vi "writeU32FIFO.vi"(8 "error in (no error)":errorcluster, 9 "Timeout":i32, 10 "Data":u32[](array[numeric]), 11 "IWriteU32FIFO in":refnum<class "IWriteU32FIFO.lvclass">) -> (0 "error out":errorcluster, 2 "ElementsRemaining":u32, 3 "IWriteU32FIFO out":refnum<class "IWriteU32FIFO.lvclass">)   [LabVIEW 2015, in "RTFPGA.lvlib" / "IWriteU32FIFO.lvclass"]
uses:
  IWriteU32FIFO.lvclass
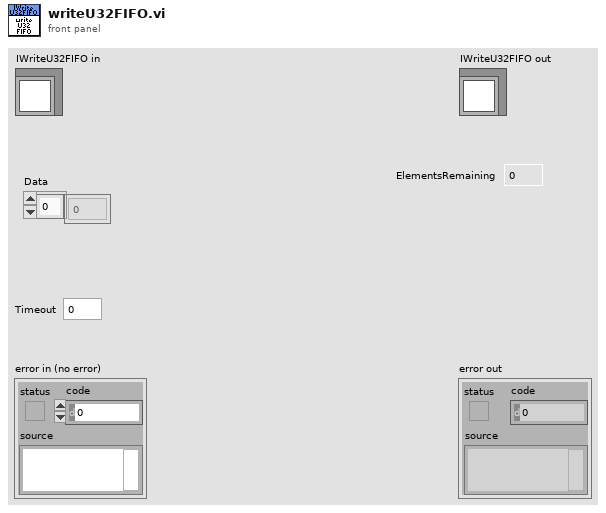
[diagram p1: front panel]
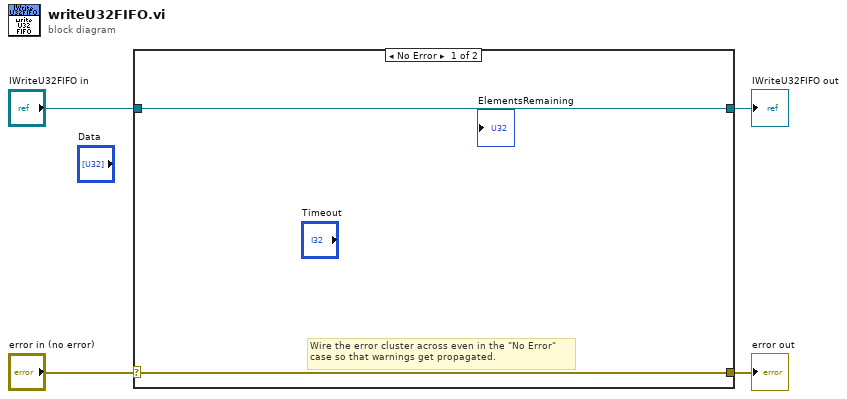
[diagram p0: block diagram]
diagram:
  n1 = case shown="No Error" "error in (no error)" {
    selector: "error in (no error)" -> [w5 w8]
    tunnel: [w5 w8] -> w3
    tunnel: [w6 w7] -> w1
    tunnel: "IWriteU32FIFO in" -> [w6 w7]
    frame No Error {
      # "Wire the error cluster across even in the \"No Error\"\ncase so that warnings get propagated."
    }
    frame Error {
    }
  }
  "error out" <- w3
  "IWriteU32FIFO out" <- w1
